vi "R3_Turn Pumps Off.vi"   [LabVIEW 2016]
uses:
  R3 pH Manual Control.ctl
  R3 Pump Manual Control.ctl
  R3Variables.lvlib
types:
  T1 = typedef "R3Variables.lvlib/R3 Pump Manual Control.ctl" = cluster{"AR Influent":bool, "AR Effluent":bool, "PR Feed":bool, "PR Decant":bool, "PR Recycle":bool, "PR Aeration":bool, "Stirring":bool}
  T2 = typedef "R3Variables.lvlib/R3 pH Manual Control.ctl" = cluster{"Acid Pump":bool, "Base Pump":bool}
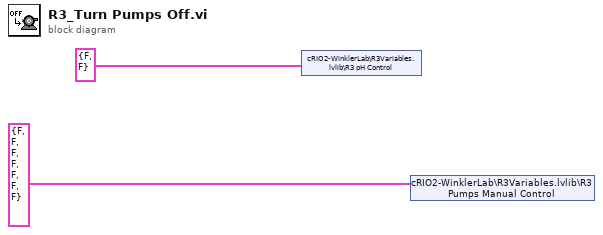
[diagram p0: block diagram]
diagram:
  n1 = shared-variable "cRIO2-WinklerLab\\R3Variables.lvlib\\R3 pH Control"(T2 {"Acid Pump"=FALSE, "Base Pump"=FALSE} ("Reactor 3 pH Control")) -> ()  [unwired: 1 in, 1 out]
  n2 = shared-variable "cRIO2-WinklerLab\\R3Variables.lvlib\\R3 Pumps Manual Control"(T1 {"AR Influent"=FALSE, "AR Effluent"=FALSE, "PR Feed"=FALSE, "PR Decant"=FALSE, "PR Recycle"=FALSE, "PR Aeration"=FALSE, "Stirring"=FALSE} ("R3 Pumps Manual Control")) -> ()  [unwired: 1 in, 1 out]
